vi "AddNewOdorsConc.vi"() -> (3 "To Add Out":string[](array[string])=["3-octanol"])   [LabVIEW 2016]
panel:
  in  "Cancel Button":bool
  in  "DOne":bool
  in  "To Add":string[](array[string])
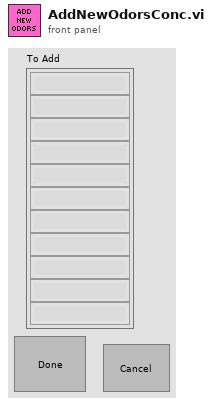
[diagram p1: front panel]
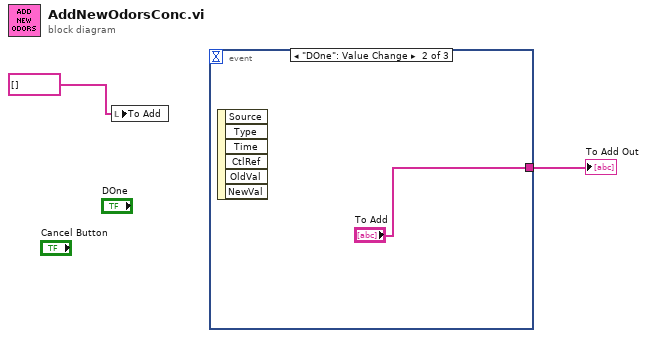
[diagram p0: block diagram]
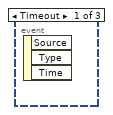
[diagram p2: hidden frame]
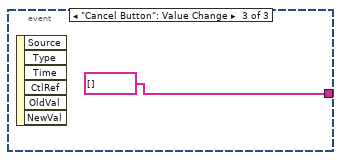
[diagram p3: hidden frame]
diagram:
  n1 = local write "To Add"(string[] []) -> ()
  n2 = event shown="[1] \"DOne\": Value Change" {
    selector: _ -> [_ _ _]
    dyn-events: _ -> [_ _ _]
    timeout: _ -> [_ _ _]
    tunnel: [_ "To Add" string[] [] ("To Add")] -> w2
    event Timeout {
      n3 = event-data() -> ()  [unwired: 1 in, 3 out]
    }
    event "DOne": Value Change {
      n4 = event-data() -> ()  [unwired: 1 in, 6 out]
    }
    event "Cancel Button": Value Change {
      n5 = event-data() -> ()  [unwired: 1 in, 6 out]
    }
  }
  "To Add Out" <- w2
